vi "Compare Calls.vi"(8 "error in (no error)":errorcluster, 9 "VI Call 2":refnum<class "VI Call.lvclass">, 10 "VI Call 1":refnum<class "VI Call.lvclass">, 11 "Tolerant Numeric Comparator In":refnum<class "Tolerant Numeric Comparator.lvclass">) -> (0 "error out":errorcluster, 1 "Description":string, 2 "Equal?":bool)   [LabVIEW 2020, in "Tolerant Numeric Comparator.lvclass"]
uses:
  Tolerant Numeric Comparator.lvclass
  Call/VI Call.lvclass
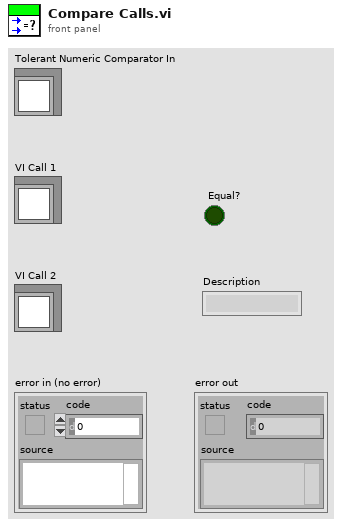
[diagram p1: front panel]
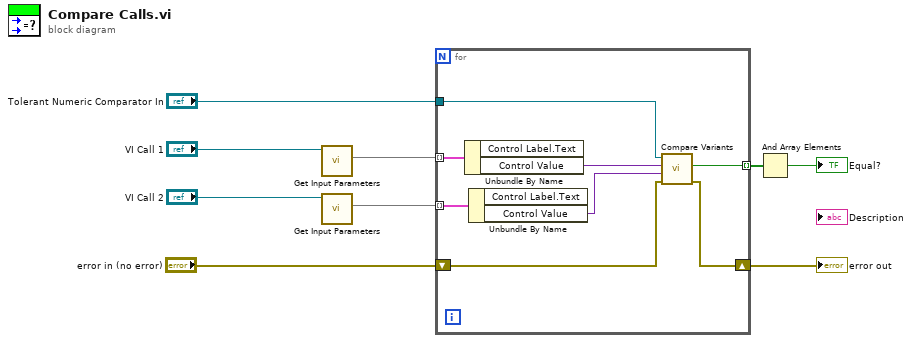
[diagram p0: block diagram]
diagram:
  n1 = call-dynamic "Get Input Parameters.vi"("VI Call In"="VI Call 1") -> ("Input Parameters"=w7:map{string, variant})  [unwired: 9 in, 1 out]
  n2 = call-dynamic "Get Input Parameters.vi"("VI Call In"="VI Call 2") -> ("Input Parameters"=w6:map{string, variant})  [unwired: 9 in, 1 out]
  n3 = for {
    tunnel: w7 -> [w17] mode=indexing
    tunnel: w6 -> [w16] mode=indexing
    tunnel: "Tolerant Numeric Comparator In" -> [w13]
    tunnel: [w12] -> w4 mode=indexing
    shift-right: [w10] -> w1
    shift-left: "error in (no error)" -> [w11]
    n4 = Unbundle By Name(w17) -> ("Control Value"=w15:variant)  [unwired: 1 out]
    n5 = Unbundle By Name(w16) -> ("Control Value"=w14:variant)  [unwired: 1 out]
    n6 = call "Compare Variants.vi"("error in (no error)"=w11, "Variant 2"=w14, "Variant 1"=w15, "Tolerant Numeric Comparator In"=w13) -> ("error out"=w10:errorcluster, "Equal?"=w12:bool)  [unwired: 5 in, 1 out]
  }
  "error out" <- w1
  n7 = And Array Elements(Boolean array=w4) -> (logical AND=→"Equal?":bool)
